vi "checkout.vi"(7 "locked by?":string, 8 "error in (no error)":errorcluster) -> (0 "error out":errorcluster, 3 "GenericImageAssembler out":refnum<class "GenericImageAssembler.lvclass">)   [LabVIEW 2010, in "GenericImageAssembler.lvclass"]
uses:
  GenericImageAssembler.lvclass
  class_data.vi
  common/classes/GenericComponent/GenericComponent/GenericComponent.lvclass
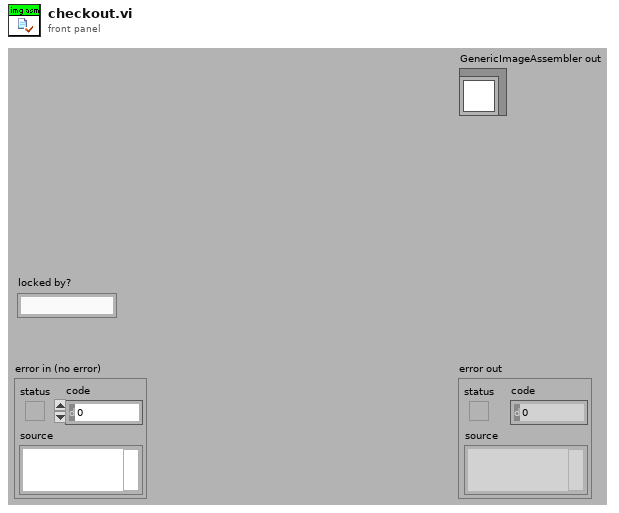
[diagram p1: front panel]
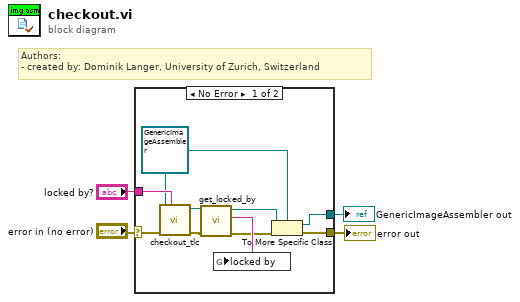
[diagram p0: block diagram]
diagram:
  # "Authors: \n- created by: Dominik Langer, University of Zurich, Switzerland"
  n1 = case shown="No Error" "error in (no error)" {
    selector: "error in (no error)" -> [w6 w15]
    tunnel: [w14 w15] -> w3
    tunnel: "locked by?" -> [w7 _]
    tunnel: [w13 _] -> w1
    frame No Error {
      w5 = refnum<class "GenericImageAssembler.lvclass"> refnum ("GenericImageAssembler.lvclass")
      n2 = call-dynamic "checkout_tlc.vi"("locked by?"=w7, "error in (no error)"=w6, "GenericToplevelComponent in"=w5) -> ("error out"=w11:errorcluster, "GenericToplevelComponent out"=w10:refnum<class "GenericToplevelComponent.lvclass">)  [unwired: 7 in]
      n3 = call "get_locked_by.vi"("error in (no error)"=w11, "GenericPlugin.lvclass in"=w10) -> ("error out"=w9:errorcluster, "locked by"=w12:string, "GenericPlugin.lvclass out"=w8:refnum<class "GenericToplevelComponent.lvclass">)  [unwired: 7 out]
      n4 = global write "class_data.vi" "locked by"(w12) -> ()
      n5 = To More Specific Class(target class=w5, reference=w8, error in=w9) -> (specific class reference=w13:refnum<class "GenericImageAssembler.lvclass">, error out=w14:errorcluster)
    }
    frame Error {
    }
  }
  "error out" <- w3
  "GenericImageAssembler out" <- w1
